vi "AutotestTester.vi"() -> ()   [LabVIEW 2020, in "Library Core.lvlib" / "Actor_Autotest.lvlib"]
uses:
  Actor_Autotest.lvlib
  Auto-test/Actor_Autotest.lvclass
  C:/Program Files (x86)/National Instruments/LabVIEW 2020/vi.lib/ActorFramework/Actor/Actor.lvclass
  Actor_Log/Actor_Log/Actor_Log/Actor_Log.lvclass
  Instrument/Class Instrument Multimeter/Class Instrument Multimeter.lvclass
  Multimeter/Multimeter Rigol DM3058/Class Multimeter Rigol DM3058.lvclass
  C:/Users/ngarcin/OneDrive - Altyor/Standard TB/Class/Multimeter/Multimeter (Default)/Class Multimeter (Default).lvclass
  Commun VI/TypeDef/Command Multimeter/Typedef Function.ctl
  Commun VI/TypeDef/Command Multimeter/Parameter Multimeter.ctl
  Multimeter/Multimeter (Default)/Class Multimeter (Default).lvclass
  Instrument/Instrument (Default)/Class Instrument (Default).lvclass
  Actor_Autotest Messages/Load_Instr_Object Msg/Load_Instr_Object Msg.lvclass/Load_Instr_Object Msg.ctl
  <vilib>/ActorFramework/Message Enqueuer/Message Enqueuer.lvclass/Message Enqueuer.ctl
  c9cca963-07f6-45a9-b5d9-d67f7eccc11f.vi
  <vilib>/ActorFramework/Message Enqueuer/Enqueue.vi
  Actor_Autotest Messages/Load_Instr_Object Msg/Load_Instr_Object Msg.lvclass
  C:/Program Files (x86)/National Instruments/LabVIEW 2020/vi.lib/ActorFramework/Message/Message.lvclass
  Actor_Autotest Messages/Register_Actor Msg/Register_Actor Msg.lvclass
  <vilib>/ActorFramework/Stop Msg/Stop Msg.lvclass
  JSON API/Variant JSON/Variant to JSON.vi
  JSON API/JSON Value/Get Item by name array.vi
  <vilib>/ActorFramework/Message Priority Queue/Priority Enqueue.vi
  JSON API/JSON Value/JSON Value.lvclass
  <vilib>/ActorFramework/Actor/Actor.lvclass
  Commun VI/Library Commun.lvlib
  JSON API/Get Polymorphic/JSON GetSet.lvlib
  JSON API/Variant JSON/Variant JSON.lvlib
panel:
  in  "AutotestName":string
  in  "Stop Button":bool
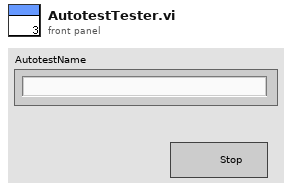
[diagram p1: front panel]
types:
  T1 = typedef "Library Commun.lvlib/Parameter Multimeter.ctl" = cluster{"Device @":refnum<visa-resource-name>, "Range":dbl, "Voltage Type":enum16{"AC", "DC"}, "Function":T2, "Class Multimeter":refnum<class "Class Multimeter (Default).lvclass">}
  T2 = typedef "Library Commun.lvlib/Typedef Function.ctl" = enum16{"Voltmeter", "Ammeter", "Continuity", "Ohmmeter", "Frequencymeter"}
  T3 = enum16{"Init", "Add Actor", "Delete Actor", "Get Actor Queue", "Get Log Actor Queue", "List all actors"}
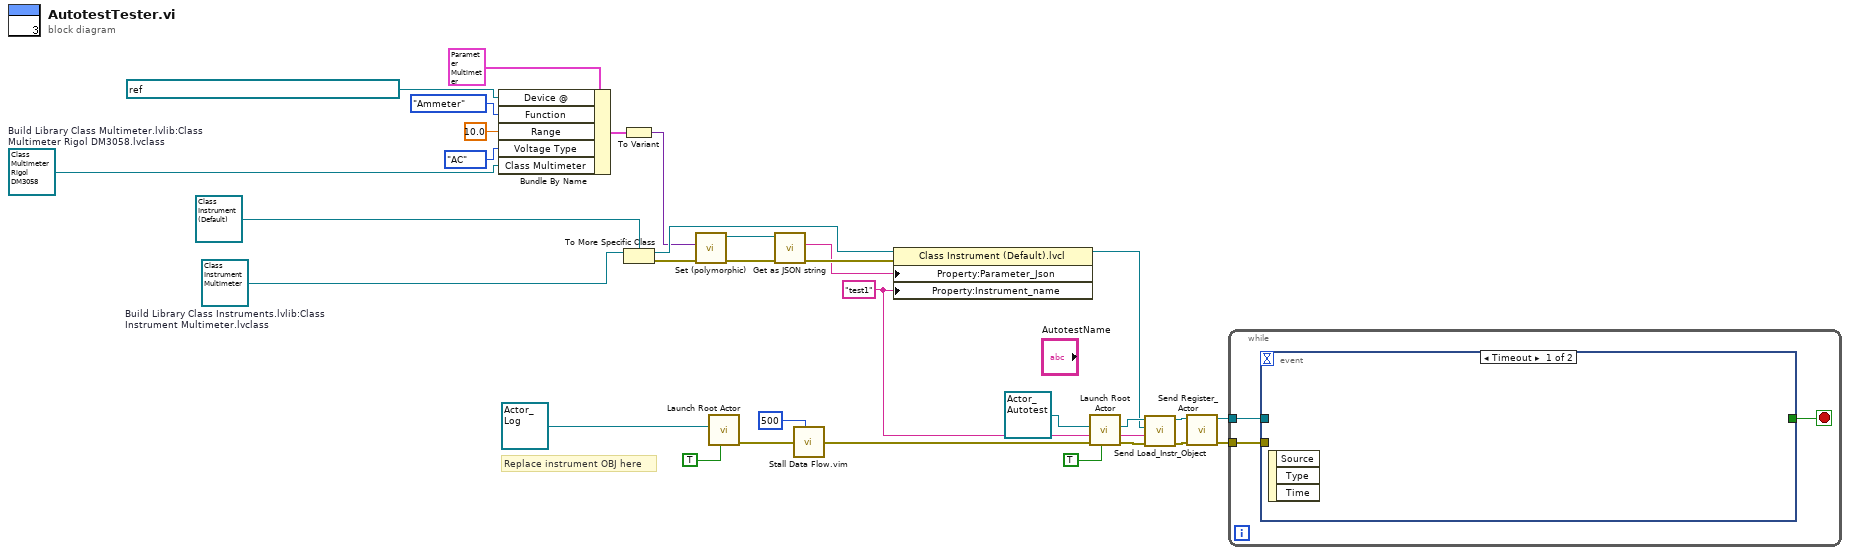
[diagram p0: block diagram]
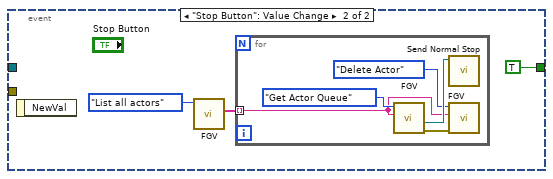
[diagram p2: hidden frame]
diagram:
  w1 = "test1" ("Instrument name")
  w14 = refnum<class "Class Multimeter Rigol DM3058.lvclass"> refnum  # Build Library Class Multimeter.lvlib:Class Multimeter Rigol DM3058.lvclass
  w13 = refnum<class "Class Instrument Multimeter.lvclass"> refnum  # Build Library Class Instruments.lvlib:Class Instrument Multimeter.lvclass
  # "Replace instrument OBJ here"
  n1 = Bundle By Name(cluster=T1 {"Device @"="", "Range"=0.0, "Voltage Type"=enum."AC", "Function"=enum."Voltmeter", "Class Multimeter"=refnum} ("Parameter"), "Device @"=refnum<visa-resource-name> "USB0::0x1AB1::0x09C4::DM3R202301192::INSTR" ("Address_Device"), "Function"=Typedef_Function."Ammeter", "Range"=10.0, "Voltage Type"=enum16{"AC", "DC"}."AC" ("Voltage_Type"), "Class Multimeter"=w14) -> (w19:T1)
  n2 = To Variant(anything=w19) -> (Variant=w6:variant)
  n3 = To More Specific Class(target class=refnum<class "Class Instrument (Default).lvclass"> refnum ("Library Instruments.lvlib:Class Instrument (Default).lvclass"), reference=w13) -> (specific class reference=w7:refnum<class "Class Instrument (Default).lvclass">, error out=w8:errorcluster)  [unwired: 1 in]
  n4 = call-poly "Set (polymorphic).vi"("error in (no error)"=w8, "Variant"=w6) -> ("error out"=w10:errorcluster, "JSON Value out"=w9:refnum<class "JSON Value.lvclass">)  [unwired: 8 in]
  n5 = call <vilib>:"Launch Root Actor.vi"("Open Actor Core front panel? (F)"=TRUE, "Actor"=refnum<class "Actor_Log.lvclass"> refnum ("Actor_Log.lvlib:Actor_Log.lvclass")) -> ("error out"=w27:errorcluster)  [unwired: 8 in, 1 out]
  n6 = call "Get as JSON string.vi"("error in (no error)"=w10, "JSON Value in"=w9) -> ("error out"=w12:errorcluster, "<JSON>"=w11:string)  [unwired: 8 in]
  n7 = call "Stall Data Flow.vim"("value in"=w27, "milliseconds to wait"=u32 500) -> ("value out"=w26:errorcluster)  [unwired: 1 out]
  n8 = property class="Class Instrument (Default).lvcl"(reference=w7, error in=w12, "Property:Parameter_Json"=w11, "Property:Instrument_name "=w1) -> (reference out=w4:refnum<class "Class Instrument (Default).lvclass">)  [unwired: 1 out]
  n9 = call <vilib>:"Launch Root Actor.vi"("Open Actor Core front panel? (F)"=TRUE, "error in (no error)"=w26, "Actor"=refnum<class "Actor_Autotest.lvclass"> refnum ("Actor_Autotest.lvlib:Actor_Autotest.lvclass")) -> ("error out"=w21:errorcluster, "Actor's Enqueuer"=w20:refnum<class "Message Enqueuer.lvclass">)  [unwired: 7 in]
  n10 = call "Send Load_Instr_Object.vi"("error in (no error)"=w21, "Instr name"=w1, "Instr obj"=w4, "Message Enqueuer"=w20) -> ("error out"=w22:errorcluster, "Message Enqueuer out"=w3:refnum<class "Message Enqueuer.lvclass">)  [unwired: 6 in]
  n11 = call "Send Register_Actor.vi"("error in (no error)"=w22, "Message Enqueuer"=w3) -> ("error out"=w24:errorcluster, "Message Enqueuer out"=w23:refnum<class "Message Enqueuer.lvclass">)  [unwired: 8 in]
  n12 = while {
    tunnel: w24 -> [w34]
    tunnel: w23 -> [w33]
    stop <- w32 stop-if-true
    n13 = event shown="[0] Timeout" {
      selector: _ -> [_ _]
      dyn-events: _ -> [_ _]
      timeout: _ -> [_ _]
      tunnel: w34 -> [_ _]
      tunnel: w33 -> [_ _]
      tunnel: [_ TRUE] -> w32
      event Timeout {
        n14 = event-data() -> ()  [unwired: 1 in, 3 out]
      }
      event "Stop Button": Value Change {
        n15 = event-data() -> ()  [unwired: 1 in, 1 out]
        n16 = call "FGV.vi"("Action"=T3."List all actors") -> ("Actor names"=w35:string[])  [unwired: 8 in, 2 out]
        n17 = for {
          tunnel: w35 -> [w38] mode=indexing
          n18 = call "FGV.vi"("Actor name"=w38, "Action"=T3."Get Actor Queue") -> ("error out"=w39:errorcluster, "Actor's Queue Out"=w41:refnum<class "Message Enqueuer.lvclass">)  [unwired: 7 in, 1 out]
          n19 = call <vilib>:"Send Normal Stop.vi"("Message Enqueuer"=w41) -> ()  [unwired: 10 in, 1 out]
          n20 = call "FGV.vi"("error in (no error)"=w39, "Actor name"=w38, "Action"=T3."Delete Actor") -> ()  [unwired: 6 in, 3 out]
        }
      }
    }
  }
